vi "Get Cal Coeffs.vi"(10 "Cal Files Path":path, 11 "Netway SNs":i32) -> (1 "Freq":cluster{dbl[], dbl[], dbl[]}, 2 "Duty":cluster{dbl[], dbl[], dbl[]}, 3 "Volts":cluster{dbl[], dbl[], dbl[]})   [LabVIEW 2010]
uses:
  <vilib>/Utility/file.llb/Read From Spreadsheet File (string).vi
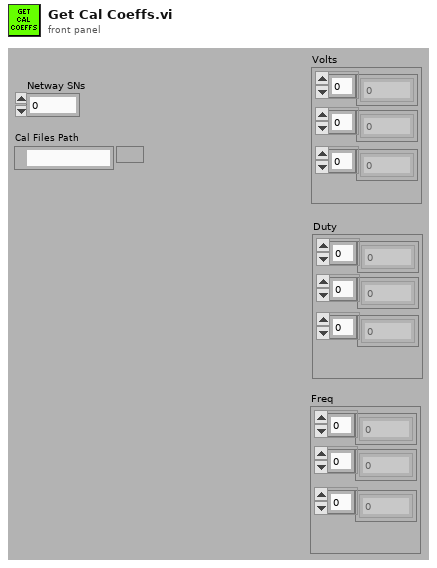
[diagram p1: front panel]
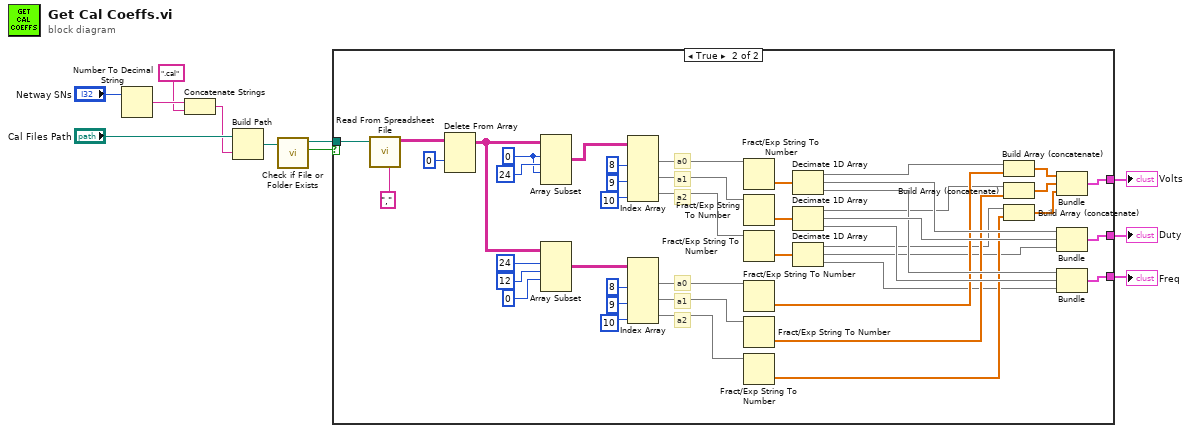
[diagram p0: block diagram]
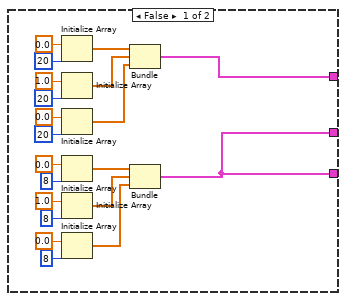
[diagram p2: hidden frame]
diagram:
  n1 = Number To Decimal String(number="Netway SNs") -> (decimal integer string=w3:string)  [unwired: 1 in]
  n2 = Concatenate Strings(w3, ".cal" ("string")) -> (w2:string)
  n3 = Build Path(base path="Cal Files Path", name or relative path=w2) -> (appended path=w11:path)
  n4 = call <vilib>:"Check if File or Folder Exists.vi"("path"=w11) -> ("file or folder exists?"=w8:bool, "dup path"=w7:path)  [unwired: 8 in, 1 out]
  n5 = case shown="True" w8 {
    tunnel: w7 -> [_ w76]
    tunnel: [w25 w60] -> w6
    tunnel: [w18 w59] -> w5
    tunnel: [w18 w58] -> w4
    frame False {
      n6 = Initialize Array(0.0 ("element"), 20 ("dimension size")) -> (w27:dbl[])
      n7 = Initialize Array(1.0 ("element"), 20 ("dimension size")) -> (w26:dbl[])
      n8 = Initialize Array(0.0 ("element"), 20 ("dimension size")) -> (w15:dbl[])
      n9 = Initialize Array(0.0 ("element"), 8 ("dimension size")) -> (w23:dbl[])
      n10 = Initialize Array(1.0 ("element"), 8 ("dimension size")) -> (w24:dbl[])
      n11 = Initialize Array(0.0 ("element"), 8 ("dimension size")) -> (w12:dbl[])
      n12 = Bundle(w27, w26, w15) -> (w25:cluster{dbl[], dbl[], dbl[]})  [unwired: 1 in]
      n13 = Bundle(w23, w24, w12) -> (w18:cluster{dbl[], dbl[], dbl[]})  [unwired: 1 in]
    }
    frame True {
      w70 = 0 ("index")
      # "a2"
      # "a2"
      # "a1"
      # "a0"
      # "a1"
      # "a0"
      n14 = call-poly <vilib>:"Read From Spreadsheet File.vi"("delimiter (\\t)"="," ("delimiter (\\t)"), "file path (dialog if empty)"=w76) -> ("all rows"=w75:string[][])  [unwired: 5 in, 4 out]
      n15 = Delete From Array(array=w75, index (row)=0) -> (array with subset deleted=w54:string[][])  [unwired: 2 in, 1 out]
      n16 = Array Subset(array=w54, index (row)=w70, length (row)=24 ("length"), index (col)=w70) -> (w69:string[][])  [unwired: 1 in]
      n17 = Array Subset(array=w54, index (row)=24 ("index"), length (row)=12 ("length"), index (col)=0 ("index")) -> (w49:string[][])  [unwired: 1 in]
      n18 = Index Array(array=w69, index (col) #1=8 ("disabled index (col)"), index (col) #2=9 ("disabled index (col)"), index (col) #3=10 ("disabled index (col)")) -> (element #1=w68:string[], element #2=w67:string[], element #3=w38:string[])  [unwired: 3 in]
      n19 = Index Array(array=w49, index (col) #1=8 ("disabled index (col)"), index (col) #2=9 ("disabled index (col)"), index (col) #3=10 ("disabled index (col)")) -> (element #1=w52:string[], element #2=w53:string[], element #3=w37:string[])  [unwired: 3 in]
      n20 = Fract/Exp String To Number(string=w68) -> (number=w66:dbl[])  [unwired: 3 in, 1 out]
      n21 = Fract/Exp String To Number(string=w67) -> (number=w65:dbl[])  [unwired: 3 in, 1 out]
      n22 = Fract/Exp String To Number(string=w38) -> (number=w41:dbl[])  [unwired: 3 in, 1 out]
      n23 = Fract/Exp String To Number(string=w52) -> (number=w47:dbl[])  [unwired: 3 in, 1 out]
      n24 = Fract/Exp String To Number(string=w53) -> (number=w45:dbl[])  [unwired: 3 in, 1 out]
      n25 = Fract/Exp String To Number(string=w37) -> (number=w35:dbl[])  [unwired: 3 in, 1 out]
      n26 = Decimate 1D Array(w66) -> (w48:dbl[], w64:dbl[], w62:dbl[])
      n27 = Decimate 1D Array(w65) -> (w46:dbl[], w63:dbl[], w61:dbl[])
      n28 = Decimate 1D Array(w41) -> (w36:dbl[], w33:dbl[], w32:dbl[])
      n29 = Build Array (concatenate)(w48, w47) -> (w44:dbl[])
      n30 = Build Array (concatenate)(w46, w45) -> (w43:dbl[])
      n31 = Build Array (concatenate)(w36, w35) -> (w34:dbl[])
      n32 = Bundle(w44, w43, w34) -> (w60:cluster{dbl[], dbl[], dbl[]})  [unwired: 1 in]
      n33 = Bundle(w64, w63, w33) -> (w59:cluster{dbl[], dbl[], dbl[]})  [unwired: 1 in]
      n34 = Bundle(w62, w61, w32) -> (w58:cluster{dbl[], dbl[], dbl[]})  [unwired: 1 in]
    }
  }
  "Volts" <- w6
  "Duty" <- w5
  "Freq" <- w4
